vi "test_read-nmea-data2.vi"() -> ()   [LabVIEW 2019] (continued)
\t\n15:09:59.33\tF9P\t$GNGSA,A,3,85,71,84,,,,,,,,,,1.28,0.68,1.09,2*08\n\t\n15:09:59.35\tF9P\t$GNGSA,A,3,36,19,11,04,09,12,,,,,,,1.28,0.68,1.09,3*0D\n\t\n15:09:59.37\tF9P\t$GNGSA,A,3,14,11,33,,,,,,,,,,1.28,0.68,1.09,4*0C\n\t\n15:09:59.39\tF9P\t$GPGSV,3,1,09,02,54,318,24,04,19,044,17,05,36,246,24,06,65,046,36,1*6E\n\t\n15:09:59.41\tF9P\t$GPGSV,3,2,09,09,45,075,29,12,24,278,21,17,34,153,22,19,53,156,26,1*68\n\t\n15:09:59.43\tF9P\t$GPGSV,3,3,09,25,12,307,17,1*5B\n\t\n15:09:59.45\tF9P\t$GPGSV,3,1,09,02,54,318,,04,19,044,,05,36,246,14,06,65,046,23,6*6E\n\t\n15:09:59.47\tF9P\t$GPGSV,3,2,09,09,45,075,16,12,24,278,,17,34,153,,19,53,156,,6*64\n\t\n15:09:59.49\tF9P\t$GPGSV,3,3,09,25,12,307,,6*5A\n\t\n15:09:59.51\tF9P\t$GLGSV,2,1,08,69,13,031,,70,73,042,,71,50,204,22,72,03,209,,1*71\n\t\n15:09:59.53\tF9P\t$GLGSV,2,2,08,77,01,327,,84,21,121,08,85,70,063,23,86,35,329,,1*7C\n\t\n15:09:59.55\tF9P\t$GLGSV,2,1,08,69,13,031,,70,73,042,,71,50,204,22,72,03,209,,3*73\n\t\n15:09:59.57\tF9P\t$GLGSV,2,2,08,77,01,327,,84,21,121,14,85,70,063,20,86,35,329,,3*70\n\t\n15:09:59.59\tF9P\t$GAGSV,2,1,08,02,09,298,14,04,66,119,25,09,31,193,20,11,71,357,22,7*7A\n\t\n15:09:59.61\tF9P\t$GAGSV,2,2,08,12,40,102,18,19,27,045,14,25,09,249,,36,25,308,20,7*75\n\t\n15:09:59.63\tF9P\t$GAGSV,2,1,08,02,09,298,,04,66,119,22,09,31,193,17,11,71,357,19,2*71\n\t\n15:09:59.65\tF9P\t$GAGSV,2,2,08,12,40,102,,19,27,045,,25,09,249,,36,25,308,,2*7E\n\t\n15:09:59.67\tF9P\t$GBGSV,1,1,03,11,50,131,20,14,87,138,22,33,60,219,26,1*49\n\t\n15:09:59.69\tF9P\t$GBGSV,1,1,03,11,50,131,21,14,87,138,22,33,60,219,,3*4E\n\t\n15:09:59.71\tF9P\t$GNGLL,3723.58468,N,12656.88727,E,061001.00,A,A*77\n\t\n15:09:59.73\tF9P\t\t\n15:09:59.75\tF9P\t\t\n15:09:59.77\tF9P\t\t\n15:09:59.79\tF9P\t\t\n15:09:59.81\tF9P\t\t\n15:09:59.83\tF9P\t\t\n15:09:59.85\tF9P\t\t\n15:09:59.87\tF9P\t\t\n15:09:59.89\tF9P\t\t\n15:09:59.91\tF9P\t\t\n15:09:59.93\tF9P\t\t\n15:09:59.95\tF9P\t\t\n15:09:59.97\tF9P\t\t\n15:09:59.99\tF9P\t\t\n15:10:00.01\tF9P\t\t\n15:10:00.03\tF9P\t\t\n15:10:00.05\tF9P\t\t\n15:10:00.07\tF9P\t\t\n15:10:00.09\tF9P\t\t\n15:10:00.11\tF9P\t\t\n15:10:00.13\tF9P\t\t\n15:10:00.15\tF9P\t\t\n15:10:00.17\tF9P\t\t\n15:10:00.19\tF9P\t\t\n15:10:00.21\tF9P\t\t\n15:10:00.23\tF9P\t\t\n15:10:00.25\tF9P\t$GNRMC,061002.00,A,3723.58425,N,12656.88664,E,2.007,232.62,250720,,,A,V*06\n\t\n15:10:00.27\tF9P\t$GNVTG,232.62,T,,M,2.007,N,3.717,K,A*23\n\t\n15:10:00.29\tF9P\t$GNGGA,061002.00,3723.58425,N,12656.88664,E,1,12,0.74,39.7,M,18.5,M,,*7F\n\t\n15:10:00.31\tF9P\t$GNGSA,A,3,12,06,19,05,17,09,04,02,,,,,1.38,0.74,1.16,1*0F\n\t\n15:10:00.33\tF9P\t$GNGSA,A,3,85,71,84,,,,,,,,,,1.38,0.74,1.16,2*0A\n\t\n15:10:00.35\tF9P\t$GNGSA,A,3,36,19,11,04,09,12,,,,,,,1.38,0.74,1.16,3*0F\n\t\n15:10:00.37\tF9P\t$GNGSA,A,3,14,11,33,,,,,,,,,,1.38,0.74,1.16,4*0E\n\t\n15:10:00.39\tF9P\t$GPGSV,3,1,09,02,54,318,31,04,19,044,18,05,36,246,25,06,65,046,30,1*62\n\t\n15:10:00.41\tF9P\t$GPGSV,3,2,09,09,45,075,33,12,24,278,22,17,34,153,24,19,53,156,26,1*66\n\t\n15:10:00.43\tF9P\t$GPGSV,3,3,09,25,12,307,16,1*5A\n\t\n15:10:00.45\tF9P\t$GPGSV,3,1,09,02,54,318,,04,19,044,,05,36,246,15,06,65,046,21,6*6D\n\t\n15:10:00.47\tF9P\t$GPGSV,3,2,09,09,45,075,15,12,24,278,,17,34,153,,19,53,156,,6*67\n\t\n15:10:00.49\tF9P\t$GPGSV,3,3,09,25,12,307,,6*5A\n\t\n15:10:00.51\tF9P\t$GLGSV,2,1,08,69,13,031,,70,73,042,,71,50,204,21,72,03,209,,1*72\n\t\n15:10:00.53\tF9P\t$GLGSV,2,2,08,77,01,327,,84,21,121,12,85,70,063,22,86,35,329,,1*76\n\t\n15:10:00.55\tF9P\t$GLGSV,2,1,08,69,13,031,,70,73,042,,71,50,204,20,72,03,209,,3*71\n\t\n15:10:00.57\tF9P\t$GLGSV,2,2,08,77,01,327,,84,21,121,07,85,70,063,17,86,35,329,,3*76\n\t\n15:10:00.59\tF9P\t$GAGSV,2,1,08,02,09,298,10,04,66,119,25,09,31,193,20,11,71,357,22,7*7E\n\t\n15:10:00.61\tF9P\t$GAGSV,2,2,08,12,40,102,17,19,27,045,15,25,09,249,,36,25,308,27,7*7C\n\t\n15:10:00.63\tF9P\t$GAGSV,2,1,08,02,09,298,,04,66,119,20,09,31,193,15,11,71,357,19,2*71\n\t\n15:10:00.65\tF9P\t$GAGSV,2,2,08,12,40,102,,19,27,045,,25,09,249,,36,25,308,,2*7E\n\t\n15:10:00.67\tF9P\t$GBGSV,1,1,03,11,50,131,19,14,87,138,23,33,60,219,26,1*42\n\t\n15:10:00.69\tF9P\t$GBGSV,1,1,03,11,50,131,19,14,87,138,22,33,60,219,,3*45\n\t\n15:10:00.71\tF9P\t$GNGLL,3723.58425,N,12656.88664,E,061002.00,A,A*7B\n\t\n15:10:00.73\tF9P\t\t\n15:10:00.75\tF9P\t\t\n15:10:00.77\tF9P\t\t\n15:10:00.79\tF9P\t\t\n15:10:00.81\tF9P\t\t\n15:10:00.83\tF9P\t\t\n15:10:00.85\tF9P\t\t\n15:10:00.87\tF9P\t\t\n15:10:00.89\tF9P\t\t\n15:10:00.91\tF9P\t\t\n15:10:00.93\tF9P\t\t\n15:10:00.95\tF9P\t\t\n15:10:00.97\tF9P\t\t\n15:10:00.99\tF9P\t\t\n15:10:01.01\tF9P\t\t\n15:10:01.03\tF9P\t\t\n15:10:01.05\tF9P\t\t\n15:10:01.07\tF9P\t\t\n15:10:01.09\tF9P\t\t\n15:10:01.11\tF9P\t\t\n15:10:01.13\tF9P\t\t\n15:10:01.15\tF9P\t\t\n15:10:01.17\tF9P\t\t\n15:10:01.19\tF9P\t\t\n15:10:01.21\tF9P\t\t\n15:10:01.23\tF9P\t\t\n15:10:01.25\tF9P\t$GNRMC,061003.00,A,3723.58379,N,12656.88621,E,1.773,,250720,,,A,V*16\n\t\n15:10:01.27\tF9P\t$GNVTG,,T,,M,1.773,N,3.283,K,A*35\n\t\n15:10:01.29\tF9P\t$GNGGA,061003.00,3723.58379,N,12656.88621,E,1,12,0.65,40.4,M,18.5,M,,*7C\n\t\n15:10:01.31\tF9P\t$GNGSA,A,3,12,06,19,05,17,09,04,02,,,,,1.20,0.65,1.00,1*01\n\t\n15:10:01.33\tF9P\t$GNGSA,A,3,85,71,84,,,,,,,,,,1.20,0.65,1.00,2*04\n\t\n15:10:01.35\tF9P\t$GNGSA,A,3,36,19,11,04,09,12,,,,,,,1.20,0.65,1.00,3*01\n\t\n15:10:01.37\tF9P\t$GNGSA,A,3,14,11,33,,,,,,,,,,1.20,0.65,1.00,4*00\n\t\n15:10:01.39\tF9P\t$GPGSV,3,1,09,02,54,318,25,04,19,044,17,05,36,246,25,06,65,046,23,1*6A\n\t\n15:10:01.41\tF9P\t$GPGSV,3,2,09,09,45,075,33,12,24,278,21,17,34,153,23,19,53,156,24,1*60\n\t\n15:10:01.43\tF9P\t$GPGSV,3,3,09,25,12,307,14,1*58\n\t\n15:10:01.45\tF9P\t$GPGSV,3,1,09,02,54,318,,04,19,044,,05,36,246,15,06,65,046,20,6*6C\n\t\n15:10:01.47\tF9P\t$GPGSV,3,2,09,09,45,075,14,12,24,278,,17,34,153,,19,53,156,,6*66\n\t\n15:10:01.49\tF9P\t$GPGSV,3,3,09,25,12,307,,6*5A\n\t\n15:10:01.51\tF9P\t$GLGSV,2,1,08,69,13,031,,70,73,042,,71,50,204,20,72,03,209,,1*73\n\t\n15:10:01.53\tF9P\t$GLGSV,2,2,08,77,01,327,,84,21,121,09,85,70,063,20,86,35,329,,1*7E\n\t\n15:10:01.55\tF9P\t$GLGSV,2,1,08,69,13,031,,70,73,042,,71,50,204,18,72,03,209,,3*7A\n\t\n15:10:01.57\tF9P\t$GLGSV,2,2,08,77,01,327,,84,21,121,10,85,70,063,16,86,35,329,,3*71\n\t\n15:10:01.59\tF9P\t$GAGSV,2,1,08,02,09,298,06,04,66,119,24,09,31,193,20,11,71,357,24,7*7E\n\t\n15:10:01.61\tF9P\t$GAGSV,2,2,08,12,40,102,16,19,27,045,17,25,09,249,,36,25,308,24,7*7C\n\t\n15:10:01.63\tF9P\t$GAGSV,2,1,08,02,09,298,,04,66,119,18,09,31,193,16,11,71,357,17,2*77\n\t\n15:10:01.65\tF9P\t$GAGSV,2,2,08,12,40,102,,19,27,045,,25,09,249,,36,25,308,,2*7E\n\t\n15:10:01.67\tF9P\t$GBGSV,1,1,03,11,50,131,18,14,87,138,23,33,60,219,25,1*40\n\t\n15:10:01.69\tF9P\t$GBGSV,1,1,03,11,50,131,17,14,87,138,21,33,60,219,,3*48\n\t\n15:10:01.71\tF9P\t$GNGLL,3723.58379,N,12656.88621,E,061003.00,A,A*75\n\t\n15:10:01.73\tF9P\t\t\n15:10:01.75\tF9P\t\t\n15:10:01.77\tF9P\t\t\n15:10:01.79\tF9P\t\t\n15:10:01.81\tF9P\t\t\n15:10:01.83\tF9P\t\t\n15:10:01.85\tF9P\t\t\n15:10:01.87\tF9P\t\t\n15:10:01.89\tF9P\t\t\n15:10:01.91\tF9P\t\t\n15:10:01.93\tF9P\t\t\n15:10:01.95\tF9P\t\t\n15:10:01.97\tF9P\t\t\n15:10:01.99\tF9P\t\t\n15:10:02.01\tF9P\t\t\n15:10:02.03\tF9P\t\t\n15:10:02.05\tF9P\t\t\n15:10:02.07\tF9P\t\t\n15:10:02.09\tF9P\t\t\n15:10:02.11\tF9P\t\t\n15:10:02.13\tF9P\t\t\n15:10:02.15\tF9P\t\t\n15:10:02.17\tF9P\t\t\n15:10:02.19\tF9P\t\t\n15:10:02.21\tF9P\t\t\n15:10:02.23\tF9P\t\t\n15:10:02.25\tF9P\t$GNRMC,061004.00,A,3723.58334,N,12656.88592,E,1.795,,250720,,,A,V*1B\n\t\n15:10:02.27\tF9P\t$GNVTG,,T,,M,1.795,N,3.325,K,A*30\n\t\n15:10:02.29\tF9P\t$GNGGA,061004.00,3723.58334,N,12656.88592,E,1,12,0.64,40.6,M,18.5,M,,*7A\n\t\n15:10:02.31\tF9P\t$GNGSA,A,3,12,06,19,05,17,09,04,02,,,,,1.19,0.64,1.00,1*0A\n\t\n15:10:02.33\tF9P\t$GNGSA,A,3,85,71,84,,,,,,,,,,1.19,0.64,1.00,2*0F\n\t\n15:10:02.35\tF9P\t$GNGSA,A,3,36,19,11,04,09,12,,,,,,,1.19,0.64,1.00,3*0A\n\t\n15:10:02.37\tF9P\t$GNGSA,A,3,14,11,33,,,,,,,,,,1.19,0.64,1.00,4*0B\n\t\n15:10:02.39\tF9P\t$GPGSV,3,1,09,02,54,318,25,04,19,044,18,05,36,246,24,06,65,046,22,1*65\n\t\n15:10:02.41\tF9P\t$GPGSV,3,2,09,09,45,075,27,12,24,278,20,17,34,153,25,19,53,156,24,1*62\n\t\n15:10:02.43\tF9P\t$GPGSV,3,3,09,25,12,307,14,1*58\n\t\n15:10:02.45\tF9P\t$GPGSV,3,1,09,02,54,318,,04,19,044,,05,36,246,15,06,65,046,18,6*67\n\t\n15:10:02.47\tF9P\t$GPGSV,3,2,09,09,45,075,13,12,24,278,,17,34,153,,19,53,156,,6*61\n\t\n15:10:02.49\tF9P\t$GPGSV,3,3,09,25,12,307,,6*5A\n\t\n15:10:02.51\tF9P\t$GLGSV,2,1,08,69,13,031,,70,73,042,,71,50,204,20,72,03,209,,1*73\n\t\n15:10:02.53\tF9P\t$GLGSV,2,2,08,77,01,327,,84,21,121,08,85,70,063,19,86,35,329,,1*75\n\t\n15:10:02.55\tF9P\t$GLGSV,2,1,08,69,13,031,,70,73,042,,71,50,204,17,72,03,209,,3*75\n\t\n15:10:02.57\tF9P\t$GLGSV,2,2,08,77,01,327,,84,21,121,10,85,70,063,16,86,35,329,,3*71\n\t\n15:10:02.59\tF9P\t$GAGSV,2,1,08,02,09,298,11,04,66,119,26,09,31,193,20,11,71,357,24,7*7A\n\t\n15:10:02.61\tF9P\t$GAGSV,2,2,08,12,40,102,16,19,27,045,19,25,09,249,,36,25,308,22,7*74\n\t\n15:10:02.63\tF9P\t$GAGSV,2,1,08,02,09,298,,04,66,119,19,09,31,193,16,11,71,357,17,2*76\n\t\n15:10:02.65\tF9P\t$GAGSV,2,2,08,12,40,102,,19,27,045,,25,09,249,,36,25,308,,2*7E\n\t\n15:10:02.67\tF9P\t$GBGSV,1,1,03,11,50,131,19,14,87,138,22,33,60,219,31,1*45\n\t\n15:10:02.69\tF9P\t$GBGSV,1,1,03,11,50,131,15,14,87,138,22,33,60,219,,3*49\n\t\n15:10:02.71\tF9P\t$GNGLL,3723.58334,N,12656.88592,E,061004.00,A,A*70\n\t\n15:10:02.73\tF9P\t\t\n15:10:02.75\tF9P\t\t\n15:10:02.77\tF9P\t\t\n15:10:02.79\tF9P\t\t\n15:10:02.81\tF9P\t\t\n15:10:02.83\tF9P\t\t\n15:10:02.85\tF9P\t\t\n15:10:02.87\tF9P\t\t\n15:10:02.89\tF9P\t\t\n15:10:02.91\tF9P\t\t\n15:10:02.93\tF9P\t\t\n15:10:02.95\tF9P\t\t\n15:10:02.97\tF9P\t\t\n15:10:02.99\tF9P\t\t\n15:10:03.01\tF9P\t\t\n15:10:03.03\tF9P\t\t\n15:10:03.05\tF9P\t\t\n15:10:03.07\tF9P\t\t\n15:10:03.09\tF9P\t\t\n15:10:03.11\tF9P\t\t\n15:10:03.13\tF9P\t\t\n15:10:03.15\tF9P\t\t\n15:10:03.17\tF9P\t\t\n15:10:03.19\tF9P\t\t\n15:10:03.21\tF9P\t\t\n15:10:03.23\tF9P\t\t\n15:10:03.25\tF9P\t$GNRMC,061005.00,A,3723.58304,N,12656.88557,E,1.382,,250720,,,A,V*12\n\t\n15:10:03.27\tF9P\t$GNVTG,,T,,M,1.382,N,2.559,K,A*3E\n\t\n15:10:03.29\tF9P\t$GNGGA,061005.00,3723.58304,N,12656.88557,E,1,12,0.72,40.6,M,18.5,M,,*76\n\t\n15:10:03.31\tF9P\t$GNGSA,A,3,12,06,19,05,17,09,04,02,,,,,1.36,0.72,1.16,1*07\n\t\n15:10:03.33\tF9P\t$GNGSA,A,3,85,71,84,,,,,,,,,,1.36,0.72,1.16,2*02\n\t\n15:10:03.35\tF9P\t$GNGSA,A,3,36,19,11,04,09,12,,,,,,,1.36,0.72,1.16,3*07\n\t\n15:10:03.37\tF9P\t$GNGSA,A,3,14,11,33,,,,,,,,,,1.36,0.72,1.16,4*06\n\t\n15:10:03.39\tF9P\t$GPGSV,3,1,09,02,54,318,26,04,19,044,18,05,36,246,26,06,65,046,25,1*63\n\t\n15:10:03.41\tF9P\t$GPGSV,3,2,09,09,45,075,29,12,24,278,19,17,34,153,26,19,53,156,23,1*62\n\t\n15:10:03.43\tF9P\t$GPGSV,3,3,09,25,12,307,15,1*59\n\t\n15:10:03.45\tF9P\t$GPGSV,3,1,09,02,54,318,,04,19,044,,05,36,246,15,06,65,046,16,6*69\n\t\n15:10:03.47\tF9P\t$GPGSV,3,2,09,09,45,075,12,12,24,278,,17,34,153,,19,53,156,,6*60\n\t\n15:10:03.49\tF9P\t$GPGSV,3,3,09,25,12,307,,6*5A\n\t\n15:10:03.51\tF9P\t$GLGSV,2,1,08,69,13,031,,70,73,042,,71,50,204,19,72,03,209,,1*79\n\t\n15:10:03.53\tF9P\t$GLGSV,2,2,08,77,01,327,,84,21,121,11,85,70,063,20,86,35,329,,1*77\n\t\n15:10:03.55\tF9P\t$GLGSV,2,1,08,69,13,031,,70,73,042,,71,50,204,20,72,03,209,,3*71\n\t\n15:10:03.57\tF9P\t$GLGSV,2,2,08,77,01,327,,84,21,121,07,85,70,063,16,86,35,329,,3*77\n\t\n15:10:03.59\tF9P\t$GAGSV,2,1,08,02,09,298,10,04,66,119,31,09,31,193,21,11,71,357,24,7*7C\n\t\n15:10:03.61\tF9P\t$GAGSV,2,2,08,12,40,102,16,19,27,045,19,25,09,249,,36,25,308,19,7*7C\n\t\n15:10:03.63\tF9P\t$GAGSV,2,1,08,02,09,298,,04,66,119,20,09,31,193,14,11,71,357,17,2*7E\n\t\n15:10:03.65\tF9P\t$GAGSV,2,2,08,12,40,102,,19,27,045,,25,09,249,,36,25,308,,2*7E\n\t\n15:10:03.67\tF9P\t$GBGSV,1,1,03,11,50,131,19,14,87,138,21,33,60,219,25,1*43\n\t\n15:10:03.69\tF9P\t$GBGSV,1,1,03,11,50,131,16,14,87,138,22,33,60,219,,3*4A\n\t\n15:10:03.71\tF9P\t$GNGLL,3723.58304,N,12656.88557,E,061005.00,A,A*7B\n\t\n15:10:03.73\tF9P\t\t\n15:10:03.75\tF9P\t\t\n15:10:03.77\tF9P\t\t\n15:10:03.79\tF9P\t\t\n15:10:03.81\tF9P\t\t\n15:10:03.83\tF9P\t\t\n15:10:03.85\tF9P\t\t\n15:10:03.87\tF9P\t\t\n15:10:03.89\tF9P\t\t\n15:10:03.91\tF9P\t\t\n15:10:03.93\tF9P\t\t\n15:10:03.95\tF9P\t\t\n15:10:03.97\tF9P\t\t\n15:10:03.99\tF9P\t\t\n15:10:04.01\tF9P\t\t\n15:10:04.03\tF9P\t\t\n15:10:04.05\tF9P\t\t\n15:10:04.07\tF9P\t\t\n15:10:04.09\tF9P\t\t\n15:10:04.11\tF9P\t\t\n15:10:04.13\tF9P\t\t\n15:10:04.15\tF9P\t\t\n15:10:04.17\tF9P\t\t\n15:10:04.19\tF9P\t\t\n15:10:04.21\tF9P\t\t\n15:10:04.23\tF9P\t\t\n15:10:04.25\tF9P\t$GNRMC,061006.00,A,3723.58291,N,12656.88483,E,2.057,245.78,250720,,,A,V*0E\n\t\n15:10:04.27\tF9P\t$GNVTG,245.78,T,,M,2.057,N,3.809,K,A*2D\n\t\n15:10:04.29\tF9P\t$GNGGA,061006.00,3723.58291,N,12656.88483,E,1,12,0.68,42.0,M,18.5,M,,*7F\n\t\n15:10:04.31\tF9P\t$GNGSA,A,3,12,06,19,05,17,09,04,02,,,,,1.26,0.68,1.06,1*0C\n\t\n15:10:04.33\tF9P\t$GNGSA,A,3,85,71,84,,,,,,,,,,1.26,0.68,1.06,2*09\n\t\n15:10:04.35\tF9P\t$GNGSA,A,3,36,19,11,04,09,12,,,,,,,1.26,0.68,1.06,3*0C\n\t\n15:10:04.37\tF9P\t$GNGSA,A,3,14,11,33,,,,,,,,,,1.26,0.68,1.06,4*0D\n\t\n15:10:04.39\tF9P\t$GPGSV,3,1,09,02,54,318,25,04,19,044,17,05,36,246,25,06,65,046,24,1*6D\n\t\n15:10:04.41\tF9P\t$GPGSV,3,2,09,09,45,075,27,12,24,278,20,17,34,153,30,19,53,156,25,1*67\n\t\n15:10:04.43\tF9P\t$GPGSV,3,3,09,25,12,307,15,1*59\n\t\n15:10:04.45\tF9P\t$GPGSV,3,1,09,02,54,318,,04,19,044,,05,36,246,16,06,65,046,15,6*69\n\t\n15:10:04.47\tF9P\t$GPGSV,3,2,09,09,45,075,13,12,24,278,,17,34,153,,19,53,156,,6*61\n\t\n15:10:04.49\tF9P\t$GPGSV,3,3,09,25,12,307,,6*5A\n\t\n15:10:04.51\tF9P\t$GLGSV,2,1,08,69,12,031,,70,73,042,,71,50,204,20,72,03,209,,1*72\n\t\n15:10:04.53\tF9P\t$GLGSV,2,2,08,77,01,327,,84,21,121,09,85,70,063,20,86,35,329,,1*7E\n\t\n15:10:04.55\tF9P\t$GLGSV,2,1,08,69,12,031,,70,73,042,,71,50,204,20,72,03,209,,3*70\n\t\n15:10:04.57\tF9P\t$GLGSV,2,2,08,77,01,327,,84,21,121,11,85,70,063,20,86,35,329,,3*75\n\t\n15:10:04.59\tF9P\t$GAGSV,2,1,08,02,09,298,07,04,66,119,27,09,31,193,21,11,71,357,26,7*7F\n\t\n15:10:04.61\tF9P\t$GAGSV,2,2,08,12,40,102,18,19,27,045,23,25,09,249,,36,25,308,19,7*7B\n\t\n15:10:04.63\tF9P\t$GAGSV,2,1,08,02,09,298,,04,66,119,21,09,31,193,,11,71,357,17,2*7A\n\t\n15:10:04.65\tF9P\t$GAGSV,2,2,08,12,40,102,,19,27,045,,25,09,249,,36,25,308,,2*7E\n\t\n15:10:04.67\tF9P\t$GBGSV,1,1,03,11,50,131,18,14,87,138,20,33,60,219,23,1*45\n\t\n15:10:04.69\tF9P\t$GBGSV,1,1,03,11,50,131,16,14,87,138,22,33,60,219,,3*4A\n\t\n15:10:04.71\tF9P\t$GNGLL,3723.58291,N,12656.88483,E,061006.00,A,A*7D\n\t\n15:10:04.73\tF9P\t\t\n15:10:04.75\tF9P\t\t\n15:10:04.77\tF9P\t\t\n15:10:04.79\tF9P\t\t\n15:10:04.81\tF9P\t\t\n15:10:04.83\tF9P\t\t\n15:10:04.85\tF9P\t\t\n15:10:04.87\tF9P\t\t\n15:10:04.89\tF9P\t\t\n15:10:04.91\tF9P\t\t\n15:10:04.93\tF9P\t\t\n15:10:04.95\tF9P\t\t\n15:10:04.97\tF9P\t\t\n15:10:04.99\tF9P\t\t\n15:10:05.01\tF9P\t\t\n15:10:05.03\tF9P\t\t\n15:10:05.05\tF9P\t\t\n15:10:05.07\tF9P\t\t\n15:10:05.09\tF9P\t\t\n15:10:05.11\tF9P\t\t\n15:10:05.13\tF9P\t\t\n15:10:05.15\tF9P\t\t\n15:10:05.17\tF9P\t\t\n15:10:05.19\tF9P\t\t\n15:10:05.21\tF9P\t\t\n15:10:05.23\tF9P\t\t\n15:10:05.25\tF9P\t$GNRMC,061007.00,A,3723.58253,N,12656.88441,E,1.799,,250720,,,A,V*1B\n\t\n15:10:05.27\tF9P\t$GNVTG,,T,,M,1.799,N,3.331,K,A*39\n\t\n15:10:05.29\tF9P\t$GNGGA,061007.00,3723.58253,N,12656.88441,E,1,12,0.68,42.6,M,18.5,M,,*78\n\t\n15:10:05.31\tF9P\t$GNGSA,A,3,12,06,19,05,17,09,04,02,,,,,1.26,0.68,1.06,1*0C\n\t\n15:10:05.33\tF9P\t$GNGSA,A,3,85,71,84,,,,,,,,,,1.26,0.68,1.06,2*09\n\t\n15:10:05.35\tF9P\t$GNGSA,A,3,36,19,11,04,09,12,,,,,,,1.26,0.68,1.06,3*0C\n\t\n15:10:05.37\tF9P\t$GNGSA,A,3,14,11,33,,,,,,,,,,1.26,0.68,1.06,4*0D\n\t\n15:10:05.39\tF9P\t$GPGSV,3,1,09,02,54,318,24,04,19,044,15,05,36,246,26,06,65,046,27,1*6E\n\t\n15:10:05.41\tF9P\t$GPGSV,3,2,09,09,45,075,28,12,24,278,19,17,34,153,24,19,53,156,24,1*66\n\t\n15:10:05.43\tF9P\t$GPGSV,3,3,09,25,12,307,15,1*59\n\t\n15:10:05.45\tF9P\t$GPGSV,3,1,09,02,54,318,,04,19,044,,05,36,246,15,06,65,046,15,6*6A\n\t\n15:10:05.47\tF9P\t$GPGSV,3,2,09,09,45,075,12,12,24,278,,17,34,153,,19,53,156,,6*60\n\t\n15:10:05.49\tF9P\t$GPGSV,3,3,09,25,12,307,,6*5A\n\t\n15:10:05.51\tF9P\t$GLGSV,2,1,08,69,12,031,,70,72,041,,71,50,204,20,72,03,209,,1*70\n\t\n15:10:05.53\tF9P\t$GLGSV,2,2,08,77,01,327,,84,21,121,13,85,70,063,21,86,35,329,,1*74\n\t\n15:10:05.55\tF9P\t$GLGSV,2,1,08,69,12,031,,70,72,041,,71,50,204,21,72,03,209,,3*73\n\t\n15:10:05.57\tF9P\t$GLGSV,2,2,08,77,01,327,,84,21,121,15,85,70,063,19,86,35,329,,3*7B\n\t\n15:10:05.59\tF9P\t$GAGSV,2,1,08,02,09,298,12,04,66,119,27,09,31,193,20,11,71,357,25,7*79\n\t\n15:10:05.61\tF9P\t$GAGSV,2,2,08,12,40,102,18,19,27,045,23,25,09,249,,36,25,308,20,7*71\n\t\n15:10:05.63\tF9P\t$GAGSV,2,1,08,02,09,298,,04,66,119,20,09,31,193,,11,71,357,17,2*7B\n\t\n15:10:05.65\tF9P\t$GAGSV,2,2,08,12,40,102,,19,27,045,,25,09,249,,36,25,308,,2*7E\n\t\n15:10:05.67\tF9P\t$GBGSV,1,1,03,11,50,131,19,14,87,138,20,33,60,219,23,1*44\n\t\n15:10:05.69\tF9P\t$GBGSV,1,1,03,11,50,131,17,14,87,138,21,33,60,219,,3*48\n\t\n15:10:05.71\tF9P\t$GNGLL,3723.58253,N,12656.88441,E,061007.00,A,A*7C\n\t\n15:10:05.73\tF9P\t\t\n15:10:05.75\tF9P\t\t\n15:10:05.77\tF9P\t\t\n15:10:05.79\tF9P\t\t\n15:10:05.81\tF9P\t\t\n15:10:05.83\tF9P\t\t\n15:10:05.85\tF9P\t\t\n15:10:05.87\tF9P\t\t\n15:10:05.89\tF9P\t\t\n15:10:05.91\tF9P\t\t\n15:10:05.93\tF9P\t\t\n15:10:05.95\tF9P\t\t\n15:10:05.97\tF9P\t\t\n15:10:05.99\tF9P\t\t\n15:10:06.01\tF9P\t\t\n15:10:06.03\tF9P\t\t\n15:10:06.05\tF9P\t\t\n15:10:06.07\tF9P\t\t\n15:10:06.09\tF9P\t\t\n15:10:06.11\tF9P\t\t\n15:10:06.13\tF9P\t\t\n15:10:06.15\tF9P\t\t\n15:10:06.17\tF9P\t\t\n15:10:06.19\tF9P\t\t\n15:10:06.21\tF9P\t\t\n15:10:06.23\tF9P\t\t\n15:10:06.25\tF9P\t$GNRMC,061008.00,A,3723.58194,N,12656.88432,E,2.008,216.95,250720,,,A,V*03\n\t\n15:10:06.27\tF9P\t$GNVTG,216.95,T,,M,2.008,N,3.720,K,A*26\n\t\n15:10:06.29\tF9P\t$GNGGA,061008.00,3723.58194,N,12656.88432,E,1,12,0.64,43.8,M,18.5,M,,*78\n\t\n15:10:06.31\tF9P\t$GNGSA,A,3,12,06,19,05,17,09,04,02,,,,,1.19,0.64,1.00,1*0A\n\t\n15:10:06.33\tF9P\t$GNGSA,A,3,85,71,84,,,,,,,,,,1.19,0.64,1.00,2*0F\n\t\n15:10:06.35\tF9P\t$GNGSA,A,3,36,19,11,04,09,12,,,,,,,1.19,0.64,1.00,3*0A\n\t\n15:10:06.37\tF9P\t$GNGSA,A,3,14,11,33,,,,,,,,,,1.19,0.64,1.00,4*0B\n\t\n15:10:06.39\tF9P\t$GPGSV,3,1,09,02,54,318,25,04,19,044,13,05,36,246,26,06,65,046,26,1*68\n\t\n15:10:06.41\tF9P\t$GPGSV,3,2,09,09,45,075,27,12,24,278,19,17,34,153,24,19,53,156,24,1*69\n\t\n15:10:06.43\tF9P\t$GPGSV,3,3,09,25,12,307,14,1*58\n\t\n15:10:06.45\tF9P\t$GPGSV,3,1,09,02,54,318,,04,19,044,,05,36,246,18,06,65,046,14,6*66\n\t\n15:10:06.47\tF9P\t$GPGSV,3,2,09,09,45,075,13,12,24,278,,17,34,153,,19,53,156,,6*61\n\t\n15:10:06.49\tF9P\t$GPGSV,3,3,09,25,12,307,,6*5A\n\t\n15:10:06.51\tF9P\t$GLGSV,2,1,08,69,12,031,,70,72,041,,71,51,205,19,72,03,209,,1*7A\n\t\n15:10:06.53\tF9P\t$GLGSV,2,2,08,77,01,327,,84,21,121,12,85,70,063,23,86,35,329,,1*77\n\t\n15:10:06.55\tF9P\t$GLGSV,2,1,08,69,12,031,,70,72,041,,71,51,205,20,72,03,209,,3*72\n\t\n15:10:06.57\tF9P\t$GLGSV,2,2,08,77,01,327,,84,21,121,15,85,70,063,20,86,35,329,,3*71\n\t\n15:10:06.59\tF9P\t$GAGSV,2,1,08,02,09,298,11,04,66,119,26,09,31,193,18,11,71,357,23,7*76\n\t\n15:10:06.61\tF9P\t$GAGSV,2,2,08,12,40,102,18,19,27,045,22,25,09,249,,36,25,308,19,7*7A\n\t\n15:10:06.63\tF9P\t$GAGSV,2,1,08,02,09,298,,04,66,119,20,09,31,193,,11,71,357,16,2*7A\n\t\n15:10:06.65\tF9P\t$GAGSV,2,2,08,12,40,102,,19,27,045,,25,09,249,,36,25,308,,2*7E\n\t\n15:10:06.67\tF9P\t$GBGSV,1,1,03,11,50,131,19,14,87,138,21,33,60,219,25,1*43\n\t\n15:10:06.69\tF9P\t$GBGSV,1,1,03,11,50,131,17,14,87,138,20,33,60,219,,3*49\n\t\n15:10:06.71\tF9P\t$GNGLL,3723.58194,N,12656.88432,E,061008.00,A,A*7F\n\t\n15:10:06.73\tF9P\t\t\n15:10:06.75\tF9P\t\t\n15:10:06.77\tF9P\t\t\n15:10:06.79\tF9P\t\t\n15:10:06.81\tF9P\t\t\n15:10:06.83\tF9P\t\t\n15:10:06.85\tF9P\t\t\n15:10:06.87\tF9P\t\t\n15:10:06.89\tF9P\t\t\n15:10:06.91\tF9P\t\t\n15:10:06.93\tF9P\t\t\n15:10:06.95\tF9P\t\t\n15:10:06.97\tF9P\t\t\n15:10:06.99\tF9P\t\t\n15:10:07.01\tF9P\t\t\n15:10:07.03\tF9P\t\t\n15:10:07.05\tF9P\t\t\n15:10:07.07\tF9P\t\t\n15:10:07.09\tF9P\t\t\n15:10:07.11\tF9P\t\t\n15:10:07.13\tF9P\t\t\n15:10:07.15\t
